vi "Global_DAQ.vi"() -> ()   [LabVIEW 2015]
panel:
  in  "Instruction":T1(ring)
  out "DAQ ready":bool
  out "Noise":dbl
  in  "QPD":cluster{"X":dbl, "Y":dbl, "intensity":dbl}
  out "Laser":bool
  out "DAQ done":bool
  out "DAQ start":bool
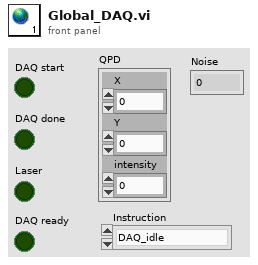
[diagram p1: front panel]
types:
  T1 = enum16{"DAQ_idle", "DAQ_initialize", "DAQ_error", "DAQ_security_stop", "DAQ_start_QPD", "DAQ_change_QPD_display", "DAQ_read_display_QPD_signal", "DAQ_QPD_init_autofocus", "DAQ_read_display_send_QPD_signal", "DAQ_close_autofocus_calibration_ramp", "DAQ_close_autofocus", "DAQ_405", "DAQ_488", "DAQ_561", "DAQ_641", "DAQ_zero_all", "DAQ_init_single_scan", "DAQ_single_scan", "DAQ_two_way_valve", "DAQ_init_merFISH", "DAQ_scan_merFISH", "DAQ_photobleaching_merFISH", "DAQ_close_merFISH", "DAQ_init_TL", "DAQ_synchro_TL", "DAQ_close_task_TL", "DAQ_close_TL", "DAQ_stop"}
diagram:
